vi "AMZ_S3_APIHLP_Multipart Upload Data FG.vi"(1 "Set?":bool, 2 "Multipart Upload Data in":T1 {"Parts"."PartNumber" min=1 max=10000}) -> (0 "Multipart Upload Data":T1 {"Parts"."PartNumber" min=1 max=10000})   [LabVIEW 2015, in "LV Interface for Amazon S3.lvlib"]
uses:
  LV Interface for Amazon S3.lvlib
  Typedefs/AMZ_S3_Multipart Upload Data.ctl
  Typedefs/AMZ_S3_Multipart Upload Part Data.ctl
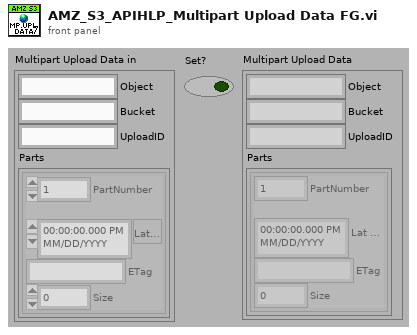
[diagram p1: front panel]
types:
  T1 = typedef "LV Interface for Amazon S3.lvlib/AMZ_S3_Multipart Upload Data.ctl" = cluster{"Object":string, "Bucket":string, "UploadID":string, "Parts":T2[]}
  T2 = typedef "LV Interface for Amazon S3.lvlib/AMZ_S3_Multipart Upload Part Data.ctl" = cluster{"PartNumber":u16, "Lat modified":timestamp, "ETag":string, "Size":u64}
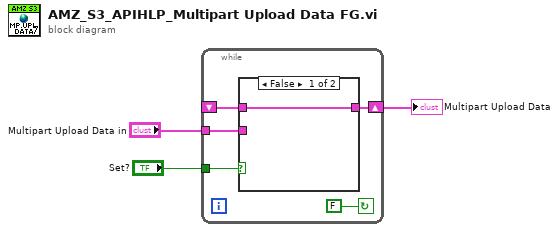
[diagram p0: block diagram]
diagram:
  n1 = while {
    tunnel: "Set?" -> [w8]
    tunnel: "Multipart Upload Data in" -> [w7]
    shift-right: [w5] -> w1
    shift-left: _ -> [w6]
    stop <- FALSE continue-if-true
    n2 = case shown="False" w8 {
      tunnel: w7 -> [_ w10]
      tunnel: w6 -> [w9 _]
      tunnel: [w9 w10] -> w5
      frame False {
      }
      frame True {
      }
    }
  }
  "Multipart Upload Data" <- w1
